vi "Tagging.vi"() -> ()   [LabVIEW 2019]
doc: "This VI demonstrates how to set and get tags that are placed on specific functions."
uses:
  <vilib>/Utility/traverseref.llb/TRef TravTarget.ctl
  <vilib>/Utility/traverseref.llb/VI Scripting - Traverse.lvlib
panel:
  in  "Tag Name":string="Example_TagName"
  # "Tagging is a way to attach arbitrary data to a GObject.  It can also be used to help identify particular objects.\n\nThis VI will open a test VI with several functions on its diagram.  It will apply a tag to one at random, then find that function based on the value of the tag. View the block diagram for more comments.\n\nWhen an object is tagged it will retain the tag forever if Is Persistent? is marked true.  If false, the tag will be removed when the VI leaves memory.\n\nIt is important to namespace any tags you are going to use.  If you set a tag with the same name as another tag on the same object, the existing information will be overwritten.  Avoid unintentionally overwriting existing tags by adding additional text to your tag name which makes it unlikely to match a tag placed by another script.  Common namespacing text follows the form COMPANYNAME_PRODUCTNAME_TAGNAME, such as 'Example_TagName' used below."
  # "Overview: Demonstrates the use of VI Scripting to assign a Tag to a random object, then uses that tag to find the object.\nInstructions:\nRun this VI. A random function in the test VI will be tagged, then this VI will find that tagged object and show its label."
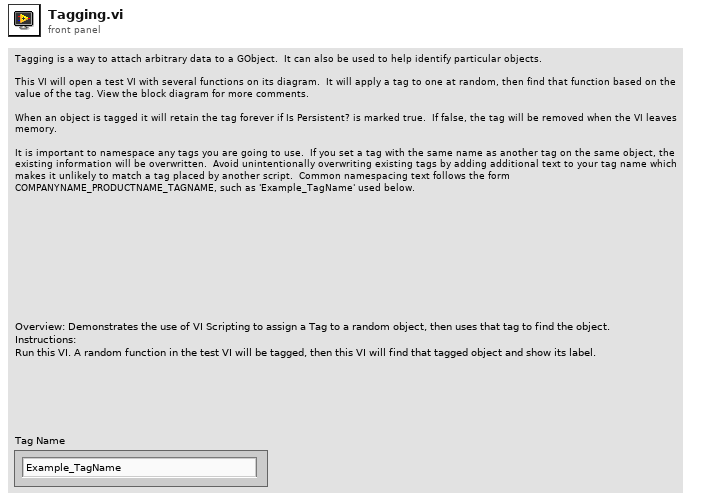
[diagram p1: front panel]
types:
  T1 = typedef "TRef TravTarget.ctl" = enum16{"FP", "BD", "Other"}
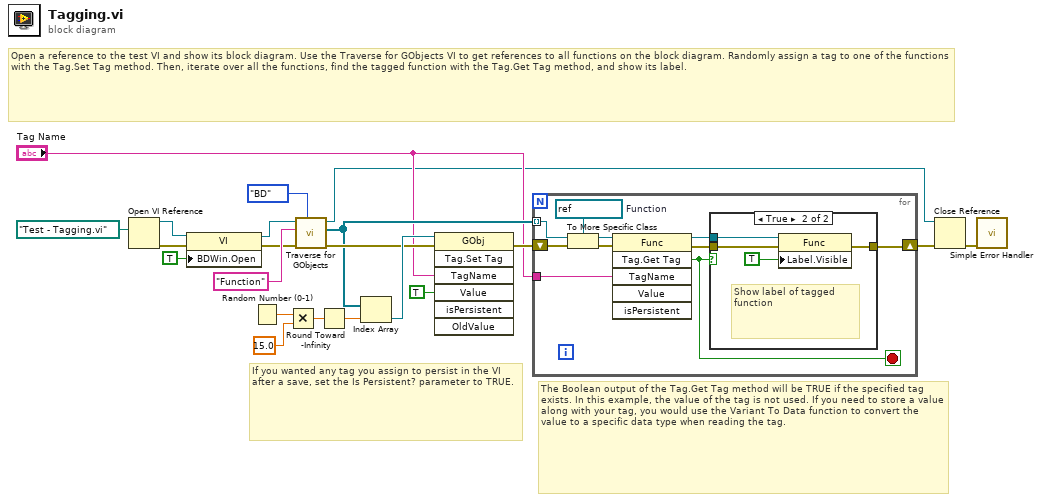
[diagram p0: block diagram]
diagram:
  # "The Boolean output of the Tag.Get Tag method will be TRUE if the specified tag exists. In this example, the value of the tag is not used. If you need to store a value along with your tag, you would use the Variant To Data function to convert the value to a specific data type when reading the tag."
  # "If you wanted any tag you assign to persist in the VI after a save, set the Is Persistent? parameter to TRUE."
  # "Open a reference to the test VI and show its block diagram. Use the Traverse for GObjects VI to get references to all functions on the block diagram. Randomly assign a tag to one of the functions with the Tag.Set Tag method. Then, iterate over all the functions, find the tagged function with the Tag.Get Tag method, and show its label."
  n1 = Open VI Reference(vi path=path "Test - Tagging.vi") -> (vi reference=w3:refnum<vi>, error out=w4:errorcluster)  [unwired: 5 in]
  n2 = property class="VI"(reference=w3, error in=w4, "BDWin.Open"=TRUE ("Block Diagram Window:Open")) -> (reference out=w5:refnum<vi>, error out=w6:errorcluster)
  n3 = Random Number (0-1)() -> (number: 0 to 1=w19:dbl)
  n4 = Multiply(x=w19, y=15.0) -> (x*y=w17:dbl)
  n5 = call <vilib>:"Traverse for GObjects.vi"("Traverse Target"=TRef_TravTarget."BD", "error in (no error)"=w6, "Class Name"="Function", "VI Refnum"=w5) -> ("error out"=w14:errorcluster, "References"=w12:refnum<vi>[], "dup VI Refnum"=w8:refnum<vi>)  [unwired: 4 in, 1 out]
  n6 = Round Toward -Infinity(1:w17) -> (0:w16:dbl)
  n7 = Index Array(array=w12, index=w16) -> (element=w15:refnum<vi>)
  n8 = invoke class="GObj" method="Tag.Set Tag"(reference=w15, error in=w14, "TagName"="Tag Name", "Value"=TRUE) -> (error out=w13:errorcluster)  [unwired: 3 in, 6 out]
  n9 = for {
    tunnel: w12 -> [w23] mode=indexing
    tunnel: "Tag Name" -> [w24]
    shift-right: [w25] -> w9
    shift-left: w13 -> [w28]
    stop <- w22 stop-if-true
    w30 = refnum<vi> refnum  # Function
    n10 = To More Specific Class(target class=w30, reference=w23, error in=w28) -> (specific class reference=w29:refnum<vi>, error out=w31:errorcluster)
    n11 = invoke class="Func" method="Tag.Get Tag"(reference=w29, error in=w31, "TagName"=w24) -> (reference out=w26:refnum<vi>, error out=w27:errorcluster, "GetTag"=w22:bool)  [unwired: 3 in, 3 out]
    n12 = case shown="True" w22 {
      tunnel: w27 -> [w32 w36]
      tunnel: w26 -> [_ w35]
      tunnel: [w32 w34] -> w25
      frame False {
      }
      frame True {
        # "Show label of tagged function"
        n13 = property class="Func"(reference=w35, error in=w36, "Label.Visible"=TRUE) -> (error out=w34:errorcluster)  [unwired: 1 out]
      }
    }
  }
  n14 = Close Reference(reference=w8, error in (no error)=w9) -> (error out=w7:errorcluster)
  n15 = call <vilib>:"Simple Error Handler.vi"("error in (no error)"=w7) -> ()  [unwired: 4 in, 5 out]
